vi "PV ActiveLine - Pirani Range Extension.vi"(7 "W/R":bool, 8 "Fehler (Eingang)":errorcluster, 9 "all gauges in":i32(ring) items=["range extension off", "range extension on"], 11 "Referenz in":refnum<visa-resource-name>) -> (0 "Cluster (Ausgang)":errorcluster, 1 "all gauges out":i32(ring) items=["range extension off", "range extension on"], 3 "Referenz out":refnum<visa-resource-name>)   [LabVIEW 2013, in "PV ActiveLine.lvlib"]
doc: "PRE - Pirani Range Extension\n\nPCR gauges only, measurement range up to 5Ч10-5 hPa.\n\nTransmit: PRE [,a]\nReceive: a\n\nPirani range extension,\na =\n0 –> Disabled (default)\n1 –> Enabled"
uses:
  <instrlib>/PV ActiveLine/PV ActiveLine.lvlib
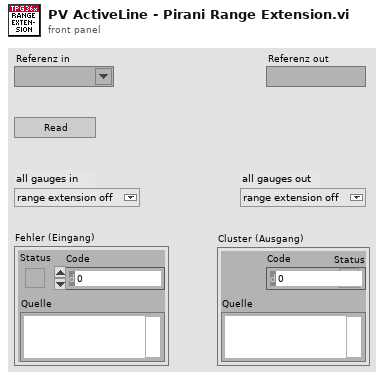
[diagram p1: front panel]
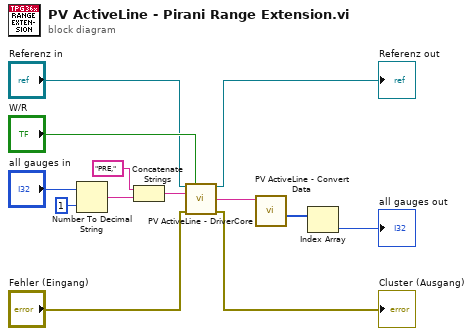
[diagram p0: block diagram]
diagram:
  n1 = Number To Decimal String(number="all gauges in", width (-)=i16 1 ("Breite (-)")) -> (decimal integer string=w6:string)
  n2 = Concatenate Strings("PRE," ("Command"), w6) -> (w8:string)
  n3 = call <instrlib>:"PV ActiveLine - DriverCore.vi"("Referenz in"="Referenz in", "Write/Read"="W/R", "Command"=w8, "Fehler (Eingang)"="Fehler (Eingang)") -> ("Referenz out"=→"Referenz out":refnum<visa-resource-name>, "String Out"=w3:string, "Cluster (Ausgang)"=→"Cluster (Ausgang)":errorcluster)  [unwired: 9 in]
  n4 = call <instrlib>:"PV ActiveLine - Convert Data.vi"("String in"=w3) -> ("Integer Out"=w2:i32[])  [unwired: 7 in, 3 out]
  n5 = Index Array(array=w2) -> (element=→"all gauges out":i32)  [unwired: 1 in]
